vi "Arduino Drive.vi"(0 "KeyInput":T1(ring)) -> (4 "Intake Out/In (T/F)":bool, 6 "Right Flower Out/In (T/F)":bool, 8 "Back Flower Out/In (T/F)":bool, 10 "Doggear Out/Engaged (T/F)":bool, 15 "Intake -1, 1 (Suck In/Suck Out)":dbl)   [LabVIEW 2013]
panel:
  out "Back Flower Activated?":bool
  out "Right Flower Activated?":bool
  out "Intake Activated?":bool
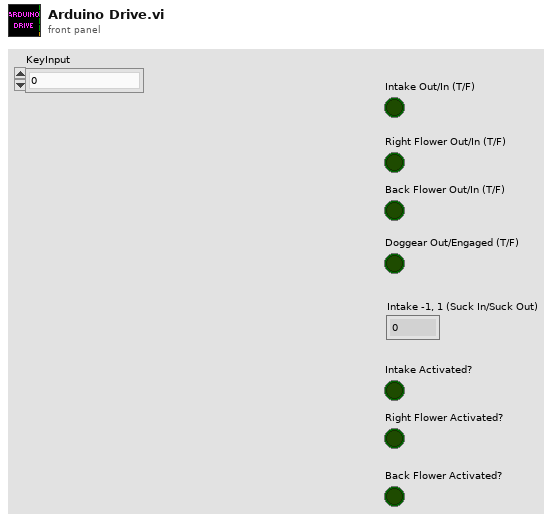
[diagram p1: front panel]
types:
  T1 = enum16{"0", "1", "2", "3", "4", "5", "6", "7", "8", "9", "A", "B", "C", "D", "E", "F", "G", "H", "I", "J", "K", "L", "M", "N", "O", "P", "Q", "R", "S", "T", "U", "V", "W", "X", "Y", "Z", "F1", "F2", "F3", "F4", "F5", "F6", "F7", "F8", "F9", "F10", "F11", "F12", "F13", "F14", "F15", "ADD", "BACK", "BACKSLASH", "CAPITAL", "COMMA", "DECIMAL", "DELETE", "DIVIDE", "DOWN", "END", "EQUALS", "ESCAPE", "GRAVE (`)", "HOME", "INSERT", "LBRACKET", "LCONTROL", "LEFT", "L ALT", "LSHIFT", "LWIN", "MINUS", "MULTIPLY", "NEXT", "NUMLOCK", "NUMPAD_0", "NUMPAD_1", "NUMPAD_2", "NUMPAD_3", "NUMPAD_4", "NUMPAD_5", "NUMPAD_6", "NUMPAD_7", "NUMPAD_8", "NUMPAD_9", "PAUSE", "PERIOD", "PRIOR (PG UP)", "RBRACKET", "RCONTROL", "RETURN", "RIGHT", "R ALT", "RSHIFT", "RWIN", "SCROLL", "SEMICOLON", "SLASH", "SPACE", "SUBTRACT", "TAB", "UP", "ENTER (num pad)", "' (quote)"}
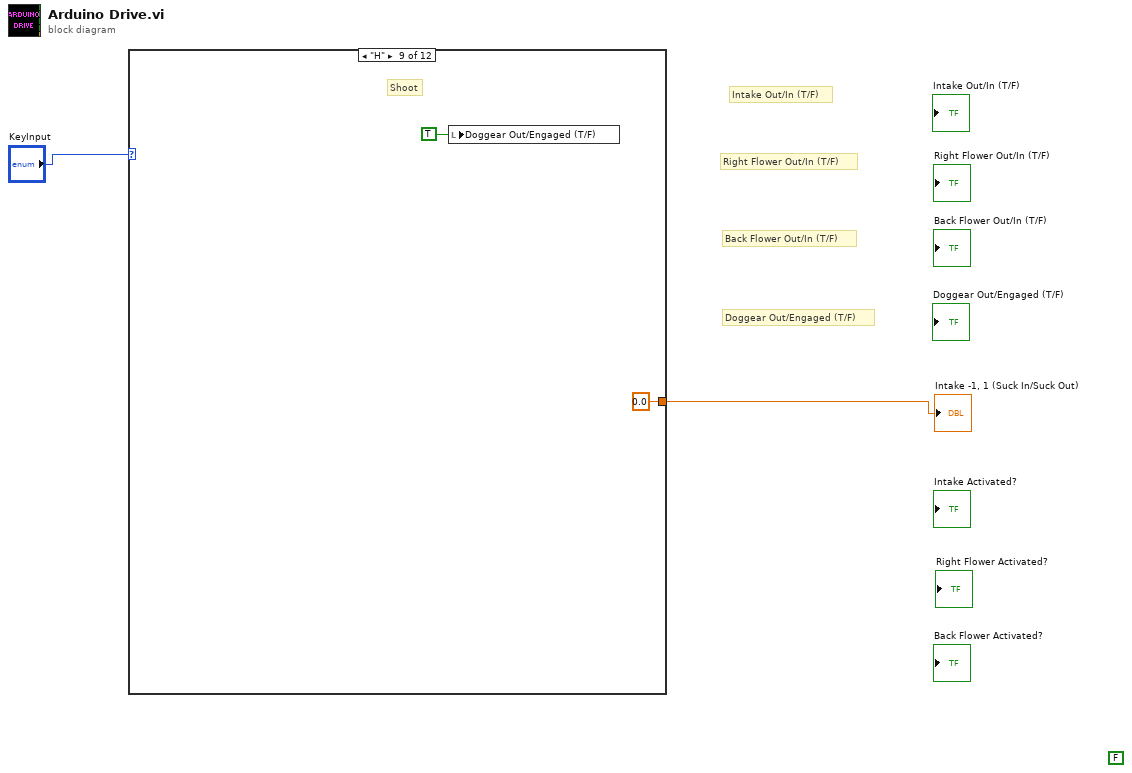
[diagram p0: block diagram]
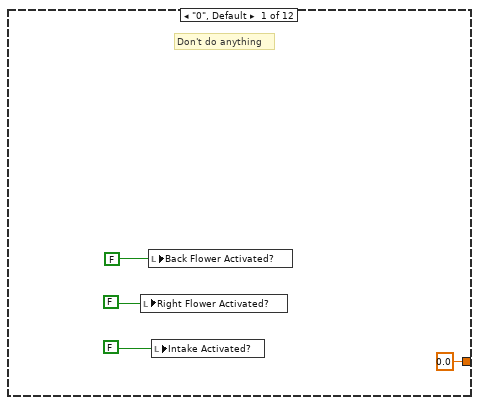
[diagram p2: hidden frame]
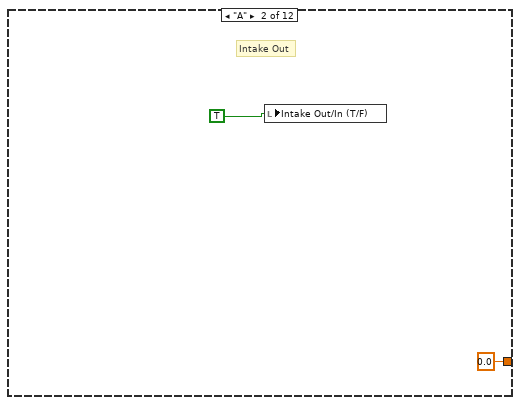
[diagram p3: hidden frame]
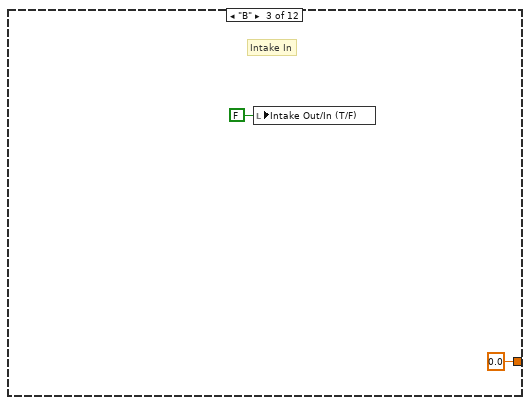
[diagram p4: hidden frame]
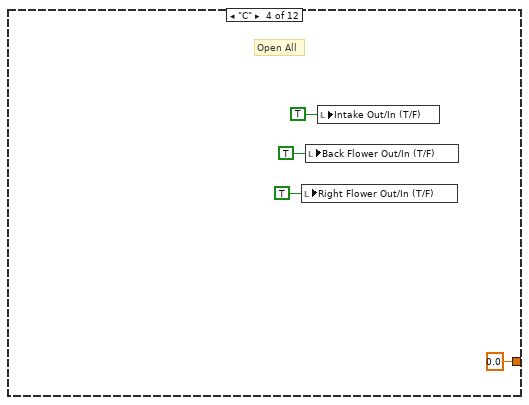
[diagram p5: hidden frame]
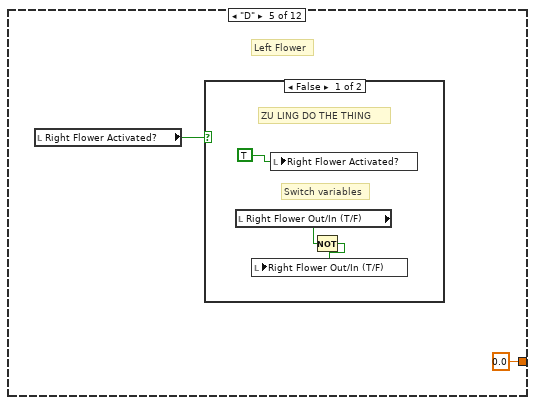
[diagram p6: hidden frame]
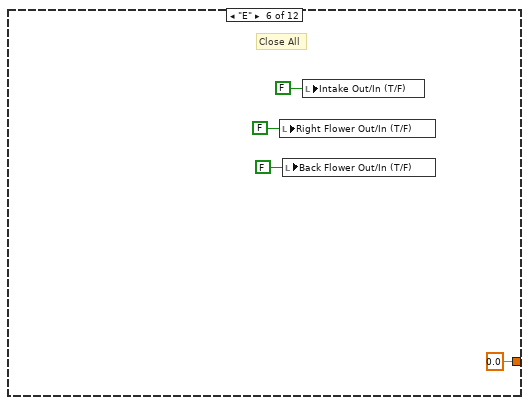
[diagram p8: hidden frame]
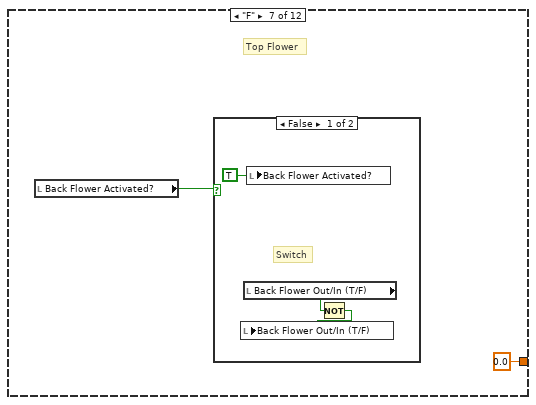
[diagram p9: hidden frame]
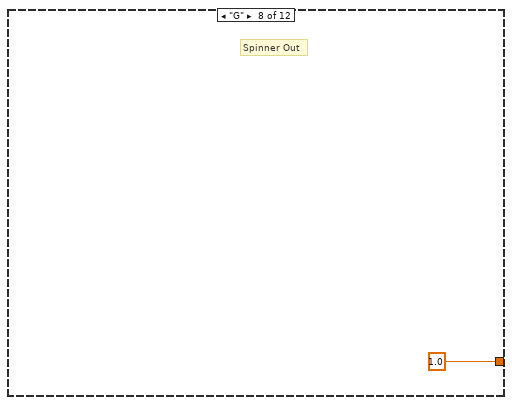
[diagram p11: hidden frame]
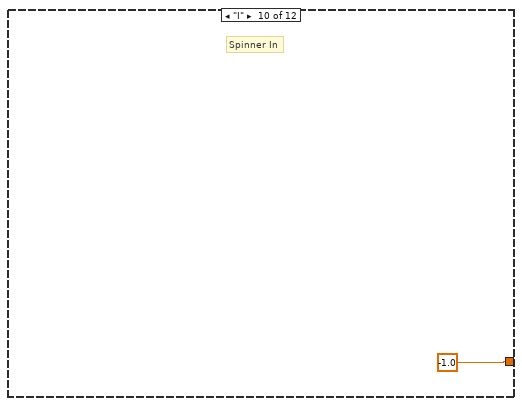
[diagram p12: hidden frame]
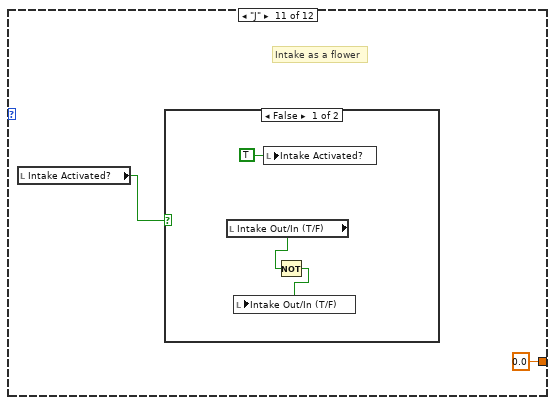
[diagram p13: hidden frame]
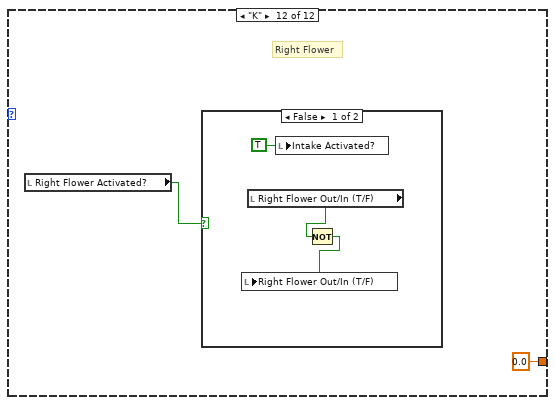
[diagram p15: hidden frame]
diagram:
  (unwired) FALSE
  # "Doggear Out/Engaged (T/F)"
  # "Back Flower Out/In (T/F)"
  # "Right Flower Out/In (T/F)"
  # "Intake Out/In (T/F)"
  n1 = case shown="\"H\"" "KeyInput" {
    tunnel: [0.0 ("Intake -1, 1 (Suck In/Suck Out)") 0.0 ("Intake -1, 1 (Suck In/Suck Out)") 0.0 ("Intake -1, 1 (Suck In/Suck Out)") 0.0 ("Intake -1, 1 (Suck In/Suck Out)") 0.0 ("Intake -1, 1 (Suck In/Suck Out)") 0.0 ("Intake -1, 1 (Suck In/Suck Out)") 0.0 ("Intake -1, 1 (Suck In/Suck Out)") 1.0 ("Intake -1, 1 (Suck In/Suck Out)") 0.0 ("Intake -1, 1 (Suck In/Suck Out)") -1.0 ("Intake -1, 1 (Suck In/Suck Out)") 0.0 ("Intake -1, 1 (Suck In/Suck Out)") 0.0 ("Intake -1, 1 (Suck In/Suck Out)")] -> w2
    frame "0", Default {
      # "Don't do anything"
      n2 = local write "Right Flower Activated?"(FALSE ("Right Flower Activated?")) -> ()
      n3 = local write "Back Flower Activated?"(FALSE ("Right Flower Activated?")) -> ()
      n4 = local write "Intake Activated?"(FALSE ("Right Flower Activated?")) -> ()
    }
    frame "A" {
      # "Intake Out"
      n5 = local write "Intake Out/In (T/F)"(TRUE) -> ()
    }
    frame "B" {
      # "Intake In"
      n6 = local write "Intake Out/In (T/F)"(FALSE ("Intake Out/In (T/F)")) -> ()
    }
    frame "C" {
      # "Open All"
      n7 = local write "Right Flower Out/In (T/F)"(TRUE ("Right Flower Out/In (T/F)")) -> ()
      n8 = local write "Back Flower Out/In (T/F)"(TRUE ("Back Flower Out/In (T/F)")) -> ()
      n9 = local write "Intake Out/In (T/F)"(TRUE ("Intake Out/In (T/F)")) -> ()
    }
    frame "D" {
      # "Left Flower"
      n10 = local read "Right Flower Activated?"() -> (w15:bool)
      n11 = case shown="False" w15 {
        frame False {
          # "Switch variables"
          # "ZU LING DO THE THING"
          n12 = local read "Right Flower Out/In (T/F)"() -> (w17:bool)
          n13 = local write "Right Flower Activated?"(TRUE) -> ()
          n14 = Not(x=w17) -> (.not. x?=w18:bool)
          n15 = local write "Right Flower Out/In (T/F)"(w18) -> ()
        }
        frame True {
          # "In a held down state"
        }
      }
    }
    frame "E" {
      # "Close All"
      n16 = local write "Right Flower Out/In (T/F)"(FALSE ("Right Flower Out/In (T/F)")) -> ()
      n17 = local write "Back Flower Out/In (T/F)"(FALSE ("Back Flower Out/In (T/F)")) -> ()
      n18 = local write "Intake Out/In (T/F)"(FALSE ("Intake Out/In (T/F)")) -> ()
    }
    frame "F" {
      # "Top Flower"
      n19 = local read "Back Flower Activated?"() -> (w24:bool)
      n20 = case shown="False" w24 {
        frame False {
          # "Switch"
          n21 = local read "Back Flower Out/In (T/F)"() -> (w27:bool)
          n22 = local write "Back Flower Activated?"(TRUE ("Back Flower Activated?")) -> ()
          n23 = Not(x=w27) -> (.not. x?=w28:bool)
          n24 = local write "Back Flower Out/In (T/F)"(w28) -> ()
        }
        frame True {
        }
      }
    }
    frame "G" {
      # "Spinner Out"
    }
    frame "H" {
      # "Shoot"
      n25 = local write "Doggear Out/Engaged (T/F)"(TRUE ("Doggear Out/Engaged (T/F)")) -> ()
    }
    frame "I" {
      # "Spinner In"
    }
    frame "J" {
      # "Intake as a flower"
      n26 = local read "Intake Activated?"() -> (w33:bool)
      n27 = case shown="False" w33 {
        frame False {
          n28 = local read "Intake Out/In (T/F)"() -> (w36:bool)
          n29 = local write "Intake Activated?"(TRUE ("Intake Activated?")) -> ()
          n30 = Not(x=w36) -> (.not. x?=w37:bool)
          n31 = local write "Intake Out/In (T/F)"(w37) -> ()
        }
        frame True {
        }
      }
    }
    frame "K" {
      # "Right Flower"
      n32 = local read "Right Flower Activated?"() -> (w38:bool)
      n33 = case shown="False" w38 {
        frame False {
          n34 = local read "Right Flower Out/In (T/F)"() -> (w41:bool)
          n35 = local write "Intake Activated?"(TRUE ("Intake Activated?")) -> ()
          n36 = Not(x=w41) -> (.not. x?=w42:bool)
          n37 = local write "Right Flower Out/In (T/F)"(w42) -> ()
        }
        frame True {
        }
      }
    }
  }
  "Intake -1, 1 (Suck In/Suck Out)" <- w2
